vi "split_averaging_filter_3cdb.vi"(4 "Reset":bool, 8 "Parameters":T1={"Order"=0, "Time constant"=0.0, "Detrend mode"=enum."Robust linear", "TD amplitude limit"=inf, "FFT filter"=TRUE, "Notch channels"=[], "LF cutoff"=0, "FD amplitude limit"=0.0}, 9 "Noise":bool, 11 "Error":cdb[](array[numeric]) format="%#_3p") -> (1 "Model":cdb[][](array[numeric]) format="%#_3p", 3 "Prediction":cdb[](array[numeric]) format="%#_3p")   [LabVIEW 2014]
uses:
  averaging_filter_params.ctl
  detrend_mode.ctl
panel:
  # "3-vector of single time sample from three signals."
  # "3-vector of predictions for the next sample, by source axis"
  # "A time domain model of the integral error on the period.  Row is source axis, columns are time step.   3 X \"Order\".   This is 2D because it has time steps as well as channels.  Synchronous with the repeat period."
  # "If true, our adaptation should be suppressed on this \"Signal\" block."
  # "This is a wrapper around split_averaging_filter_cdb.vi which adapts it to filter 3 scalar signals.  Arguments are  passed through with some data shuffling."
  # "Reset clears state to zeroes.  Filter must then settle to the steady-state output (multiple time constants)."
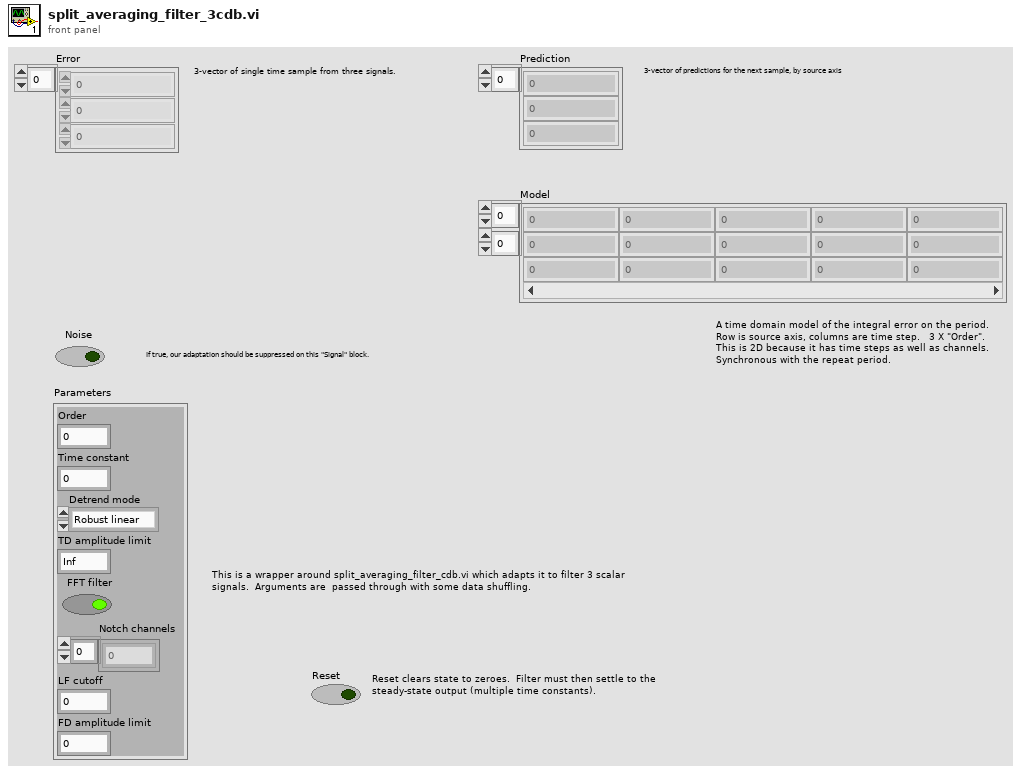
[diagram p1: front panel]
types:
  T1 = typedef "averaging_filter_params.ctl" = cluster{"Order":i32, "Time constant":dbl, "Detrend mode":T2, "TD amplitude limit":dbl, "FFT filter":bool, "Notch channels":i32[], "LF cutoff":i32, "FD amplitude limit":dbl}
  T2 = typedef "detrend_mode.ctl" = enum16{"Zero mean", "Linear", "Robust linear"}
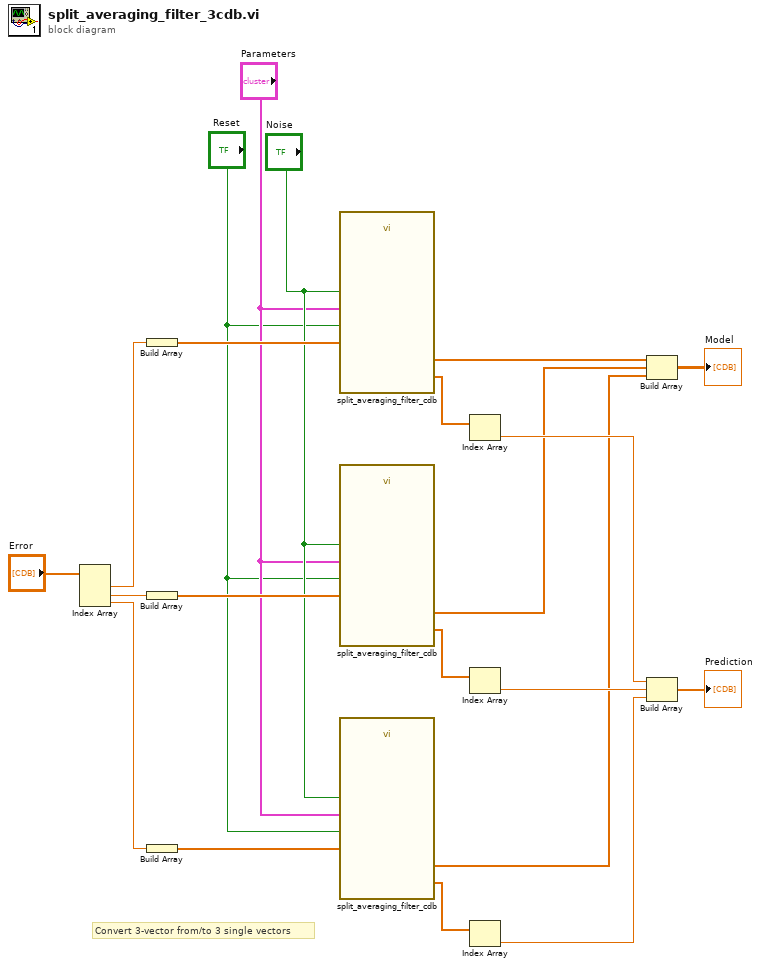
[diagram p0: block diagram]
diagram:
  # "Convert 3-vector from/to 3 single vectors"
  n1 = Index Array(array="Error") -> (element #1=w12:cdb, element #2=w11:cdb, element #3=w10:cdb)  [unwired: 3 in]
  n2 = Build Array(w12) -> (w8:cdb[])
  n3 = Build Array(w11) -> (w9:cdb[])
  n4 = Build Array(w10) -> (w7:cdb[])
  n5 = call "split_averaging_filter_cdb.vi"("Reset"="Reset", "Parameters"="Parameters", "Noise"="Noise", "Error"=w8) -> ("Model"=w3:cdb[], "Prediction"=w21:cdb[])  [unwired: 6 in]
  n6 = call "split_averaging_filter_cdb.vi"("Reset"="Reset", "Parameters"="Parameters", "Noise"="Noise", "Error"=w9) -> ("Model"=w2:cdb[], "Prediction"=w20:cdb[])  [unwired: 6 in]
  n7 = call "split_averaging_filter_cdb.vi"("Reset"="Reset", "Parameters"="Parameters", "Noise"="Noise", "Error"=w7) -> ("Model"=w1:cdb[], "Prediction"=w19:cdb[])  [unwired: 6 in]
  n8 = Index Array(array=w21) -> (element=w18:cdb)  [unwired: 1 in]
  n9 = Index Array(array=w20) -> (element=w17:cdb)  [unwired: 1 in]
  n10 = Index Array(array=w19) -> (element=w16:cdb)  [unwired: 1 in]
  n11 = Build Array(w3, w2, w1) -> (→"Model":cdb[][])
  n12 = Build Array(w18, w17, w16) -> (→"Prediction":cdb[])
